vi "decrypt.vi"(0 "HGF_GPG":refnum<class "HGF_GPG.lvclass">, 1 "options file":path, 2 "keyringfile":path, 3 "Sec keyringfile":path, 4 "string in":string, 5 "error in (no error)":errorcluster, 7 "password":string, 8 "Trust DB":path) -> (10 "dup Trust DB":path, 11 "success":bool=TRUE, 13 "data error":bool, 14 "dup HGF_GPG":refnum<class "HGF_GPG.lvclass">, 15 "dup options file":path, 16 "dup keyringfile":path, 17 "dup Sec keyringfile":path, 18 "String":string, 19 "error out":errorcluster)   [LabVIEW 2012, in "HGF_GPG.lvlib" / "HGF_GPG.lvclass"]
doc: "Decrypt a string.\nIf no password is set, the private password will be used."
uses:
  HGF_GPG.lvclass
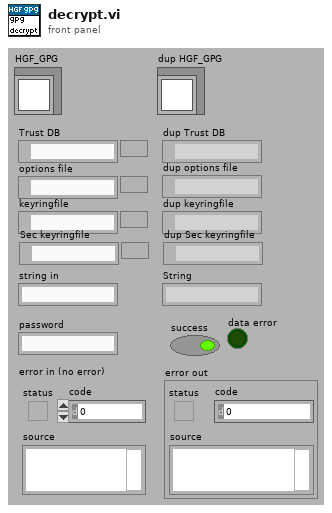
[diagram p1: front panel]
types:
  T1 = enum16{"open", "replace", "create", "open or create", "replace or create", "replace or create with confirmation"}
  T2 = enum16{"encrypt", "decrypt", "sign", "verify", "sign & encrypt", "verify & decrypt"}
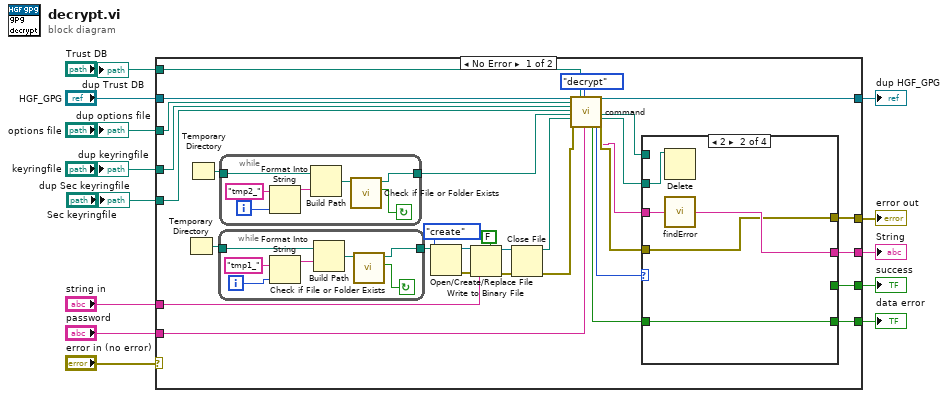
[diagram p0: block diagram]
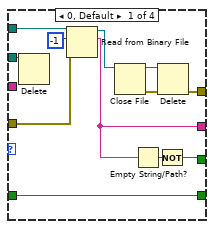
[diagram p2: hidden frame]
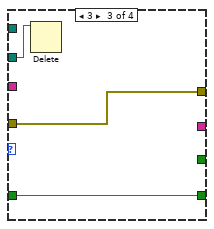
[diagram p3: hidden frame]
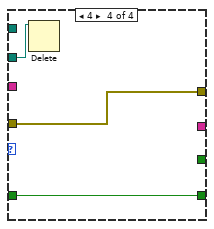
[diagram p4: hidden frame]
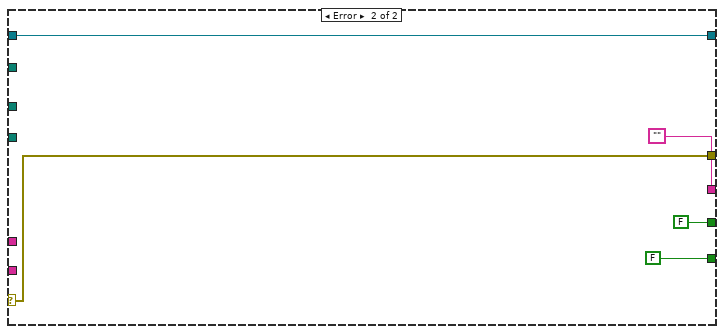
[diagram p5: hidden frame]
diagram:
  n1 = case shown="No Error" "error in (no error)" {
    selector: "error in (no error)" -> [_ w85]
    tunnel: [w43 w86] -> w11
    tunnel: "HGF_GPG" -> [w44 w86]
    tunnel: "password" -> [w24 _]
    tunnel: "string in" -> [w27 _]
    tunnel: [w38 ""] -> w8
    tunnel: [w37 w85] -> w7
    tunnel: [w29 FALSE] -> w6
    tunnel: [w28 FALSE ("data error")] -> w5
    tunnel: "options file" -> [w21 _]
    tunnel: "keyringfile" -> [w20 _]
    tunnel: "Sec keyringfile" -> [w15 _]
    tunnel: "Trust DB" -> [w14 _]
    frame No Error {
      n2 = Temporary Directory() -> (w36:path)
      n3 = Temporary Directory() -> (w35:path)
      n4 = while {
        tunnel: w36 -> [w81]
        tunnel: [w79] -> w32
        i -> [w75]
        stop <- w78 continue-if-true
        n5 = Format Into String(initial string="tmp1_" ("name or relative path"), w75) -> (resulting string=w77:string)  [unwired: 2 in, 1 out]
        n6 = Build Path(base path=w81, name or relative path=w77) -> (appended path=w80:path)
        n7 = call <vilib>:"Check if File or Folder Exists.vi"("path"=w80) -> ("file or folder exists?"=w78:bool, "dup path"=w79:path)  [unwired: 1 in, 8 out]
      }
      n8 = while {
        tunnel: w35 -> [w74]
        tunnel: [w72] -> w22
        i -> [w69]
        stop <- w71 continue-if-true
        n9 = Format Into String(initial string="tmp2_" ("name or relative path"), w69) -> (resulting string=w70:string)  [unwired: 2 in, 1 out]
        n10 = Build Path(base path=w74, name or relative path=w70) -> (appended path=w73:path)
        n11 = call <vilib>:"Check if File or Folder Exists.vi"("path"=w73) -> ("file or folder exists?"=w71:bool, "dup path"=w72:path)  [unwired: 1 in, 8 out]
      }
      n12 = Open/Create/Replace File(file path (use dialog)=w32, operation (0:open)=T1."create") -> (refnum out=w31:refnum<file>, error out=w33:errorcluster)  [unwired: 1 in, 4 out]
      n13 = Write to Binary File(file (use dialog)=w31, data=w27, error in=w33, 5:FALSE ("prepend array or string size? (T)")) -> (refnum out=w41:refnum<file>, error out=w42:errorcluster)  [unwired: 3 out]
      n14 = Close File(refnum=w41, error in=w42) -> (path=w23:path, error out=w26:errorcluster)
      n15 = call-dynamic "command.vi"("HGF_GPG"=w44, "options file"=w21, "keyringfile"=w20, "Sec keyringfile"=w15, "targetfile"=w22, "sourcefile"=w23, "error in (no error)"=w26, "Trust DB"=w14, "task"=T2."decrypt", "password"=w24) -> ("data error"=w39:bool, "return code"=w19:i32, "dup HGF_GPG"=w43:refnum<class "HGF_GPG.lvclass">, "dup targetfile"=w17:path, "dup sourcefile"=w18:path, "standard error"=w16:string, "error out"=w40:errorcluster)  [unwired: 3 in, 8 out]
      n16 = case shown="2" w19 {
        tunnel: w18 -> [w49 w60 w64 w67]
        tunnel: w40 -> [w52 w59 w63 w66]
        tunnel: w39 -> [w51 w58 w62 w65]
        tunnel: [w47 w61 _ _] -> w38
        tunnel: [w53 w59 w63 w66] -> w37
        tunnel: [w45 _ _ _] -> w29
        tunnel: [w51 w58 w62 w65] -> w28
        tunnel: w17 -> [w48 _ _ _]
        tunnel: w16 -> [_ w57 _ _]
        frame 0, Default {
          n17 = Delete(path (use dialog)=w49) -> ()  [unwired: 1 in, 6 out]
          n18 = Read from Binary File(8:w52, 10:-1 ("count (1)"), 11:w48) -> (2:w47:string, 3:w56:refnum<file>)  [unwired: 5 out]
          n19 = Close File(refnum=w56) -> (path=w54:path, error out=w55:errorcluster)  [unwired: 1 in]
          n20 = Empty String/Path?(string/path=w47) -> (empty?=w46:bool)
          n21 = Not(x=w46) -> (.not. x?=w45:bool)
          n22 = Delete(path (use dialog)=w54, error in=w55) -> (error out=w53:errorcluster)  [unwired: 5 out]
        }
        frame 2 {
          n23 = Delete(path (use dialog)=w60) -> ()  [unwired: 1 in, 6 out]
          n24 = call "findError.vi"("error string in"=w57) -> ("error out"=w61:string)
        }
        frame 3 {
          n25 = Delete(path (use dialog)=w64) -> ()  [unwired: 1 in, 6 out]
        }
        frame 4 {
          n26 = Delete(path (use dialog)=w67) -> ()  [unwired: 1 in, 6 out]
        }
      }
    }
    frame Error {
    }
  }
  "dup HGF_GPG" <- w11
  "String" <- w8
  "error out" <- w7
  "success" <- w6
  "data error" <- w5
  "dup options file" <- "options file"
  "dup keyringfile" <- "keyringfile"
  "dup Sec keyringfile" <- "Sec keyringfile"
  "dup Trust DB" <- "Trust DB"
